vi "GITGetRoot.vi"(8 "error in":errorcluster, 10 "RepoROOT":path) -> (0 "error out":errorcluster, 2 "path":path)   [LabVIEW 2020, in "CICD.lvlib"]
doc: "Returns the root of the git directory providing the current code is being run from a GIT tracked project.\nRequires local GIT installation."
uses:
  CICD.lvlib
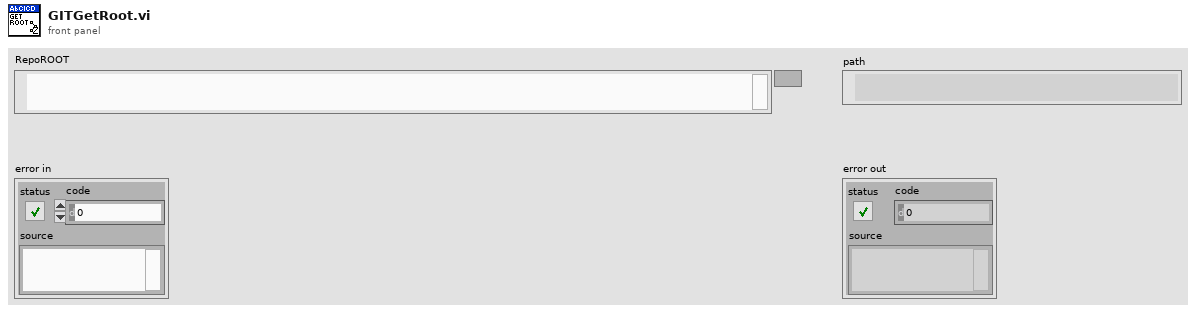
[diagram p1: front panel]
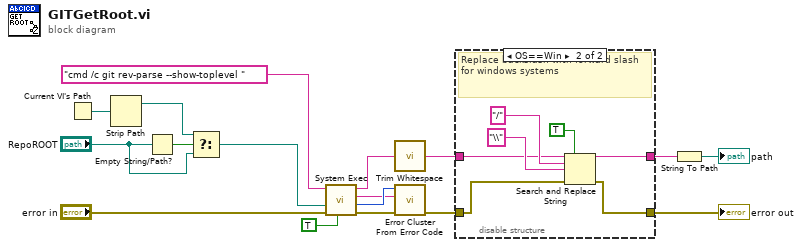
[diagram p0: block diagram]
diagram:
  n1 = Current VI's Path() -> (path=w4:path)
  n2 = Strip Path(path=w4) -> (stripped path=w3:path)  [unwired: 1 out]
  n3 = Empty String/Path?(string/path="RepoROOT") -> (empty?=w5:bool)
  n4 = Select(t=w3, s=w5, f="RepoROOT") -> (s? t:f=w1:path)
  n5 = call <vilib>:"System Exec.vi"("run minimized? (F)"=TRUE, "error in (no error)"="error in", "working directory"=w1, "command line"="cmd /c git rev-parse --show-toplevel ") -> ("error out"=w16:errorcluster, "return code"=w10:i32, "standard error"=w9:string, "standard output"=w12:string)  [unwired: 4 in]
  n6 = call <vilib>:"Trim Whitespace.vi"("string"=w12) -> ("trimmed string"=w7:string)  [unwired: 1 in]
  n7 = call <vilib>:"Error Cluster From Error Code.vi"("error in (no error)"=w16, "error message (\"\")"=w9, "error code (0)"=w10) -> ("error out"=w15:errorcluster)  [unwired: 6 in]
  n8 = disable-structure shown="OS==Win" {
    disable-tunnel: w7 -> [w18 w21]
    disable-tunnel: [w18 w20] -> w6
    disable-tunnel: w15 -> [w19 w26]
    disable-tunnel: [w19 w25] -> w14
    frame condition #0 {
    }
    frame condition #1 (active) {
      # "Replace backslash with forward slash for windows systems"
      n9 = Search and Replace String(replace all?=TRUE ("replace all? (F)"), input string=w21, search string="/", replace string="\\" ("replace string (\"\")"), error in=w26) -> (result string=w20:string, error out=w25:errorcluster)  [unwired: 3 in, 2 out]
    }
  }
  "error out" <- w14
  n10 = String To Path(string=w6) -> (path=→"path":path)
